vi "SERIAL_IntegrationControlGlobal.vi"(9 "ResetDisplacement":bool=TRUE, 10 "ResetYaw":bool=TRUE, 11 "Set":bool=TRUE) -> (1 "ResetDisplacement":bool=TRUE, 2 "ResetYaw":bool=TRUE)   [LabVIEW 2014, in "navX-MXP IMU.lvlib"]
uses:
  navX-MXP IMU.lvlib
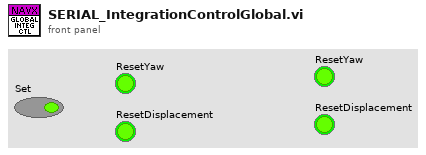
[diagram p1: front panel]
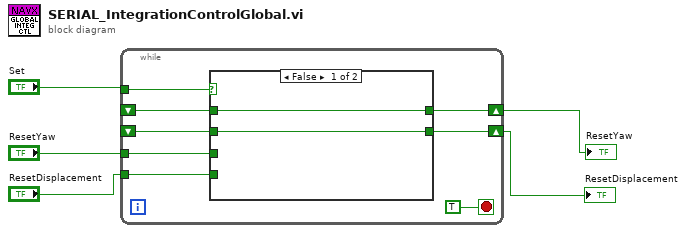
[diagram p0: block diagram]
diagram:
  n1 = while {
    shift-right: [w7] -> w1
    shift-left: _ -> [w11]
    tunnel: "Set" -> [w12]
    shift-right: [w8] -> w2
    shift-left: _ -> [w6]
    tunnel: "ResetYaw" -> [w10]
    tunnel: "ResetDisplacement" -> [w9]
    stop <- TRUE stop-if-true
    n2 = case shown="False" w12 {
      tunnel: w11 -> [w14 _]
      tunnel: w10 -> [_ w17]
      tunnel: w9 -> [_ w16]
      tunnel: [w15 w17] -> w8
      tunnel: [w14 w16] -> w7
      tunnel: w6 -> [w15 _]
      frame False {
      }
      frame True {
      }
    }
  }
  "ResetYaw" <- w2
  "ResetDisplacement" <- w1
